vi "pp2_logLoad_trialStringArray.vi"(9 "Input string array":string[](array[string])) -> (2 "Was TRIAL?":bool, 3 "Trial in":T1={"Trial Type Number"=1, "Trial Type"=enum."GO", "Trial Weight"=100, "Shock (mA)"=0.3, "Duration (ms)"=0.25, "Sound Type"=enum."04 FM Sweep", "Stim P1"=4000.0, "Stim P2"=0.0, "Stim P3"=0.0, "Stim P4"=2000.0} {"Shock (mA)" min=-1.0 max=5.0; "Trial Weight" step=1; "Duration (ms)" min=0.0 max=1.0; "Trial Type Number" min=1 max=256 step=1})   [LabVIEW 2013]
uses:
  pp2_CTL_Trial.ctl
  pp2_CTL_TrialType.ctl
  labolabo2/waveforms/WFTypes.ctl
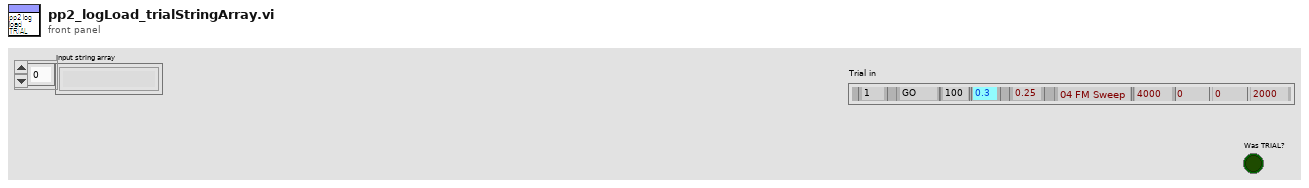
[diagram p1: front panel]
types:
  T1 = typedef "pp2_CTL_Trial.ctl" = cluster{"Trial Type Number":i16, "Trial Type":T2, "Trial Weight":u32, "Shock (mA)":dbl, "Duration (ms)":dbl, "Sound Type":T3, "Stim P1":dbl, "Stim P2":dbl, "Stim P3":dbl, "Stim P4":dbl}
  T2 = typedef "pp2_CTL_TrialType.ctl" = enum16{"OFF", "GO", "NOGO", "TEST"}
  T3 = typedef "WFTypes.ctl" = enum16{"00 NULL", "01 DC", "02 Noise", "03 Pure Tone", "04 FM Sweep"}
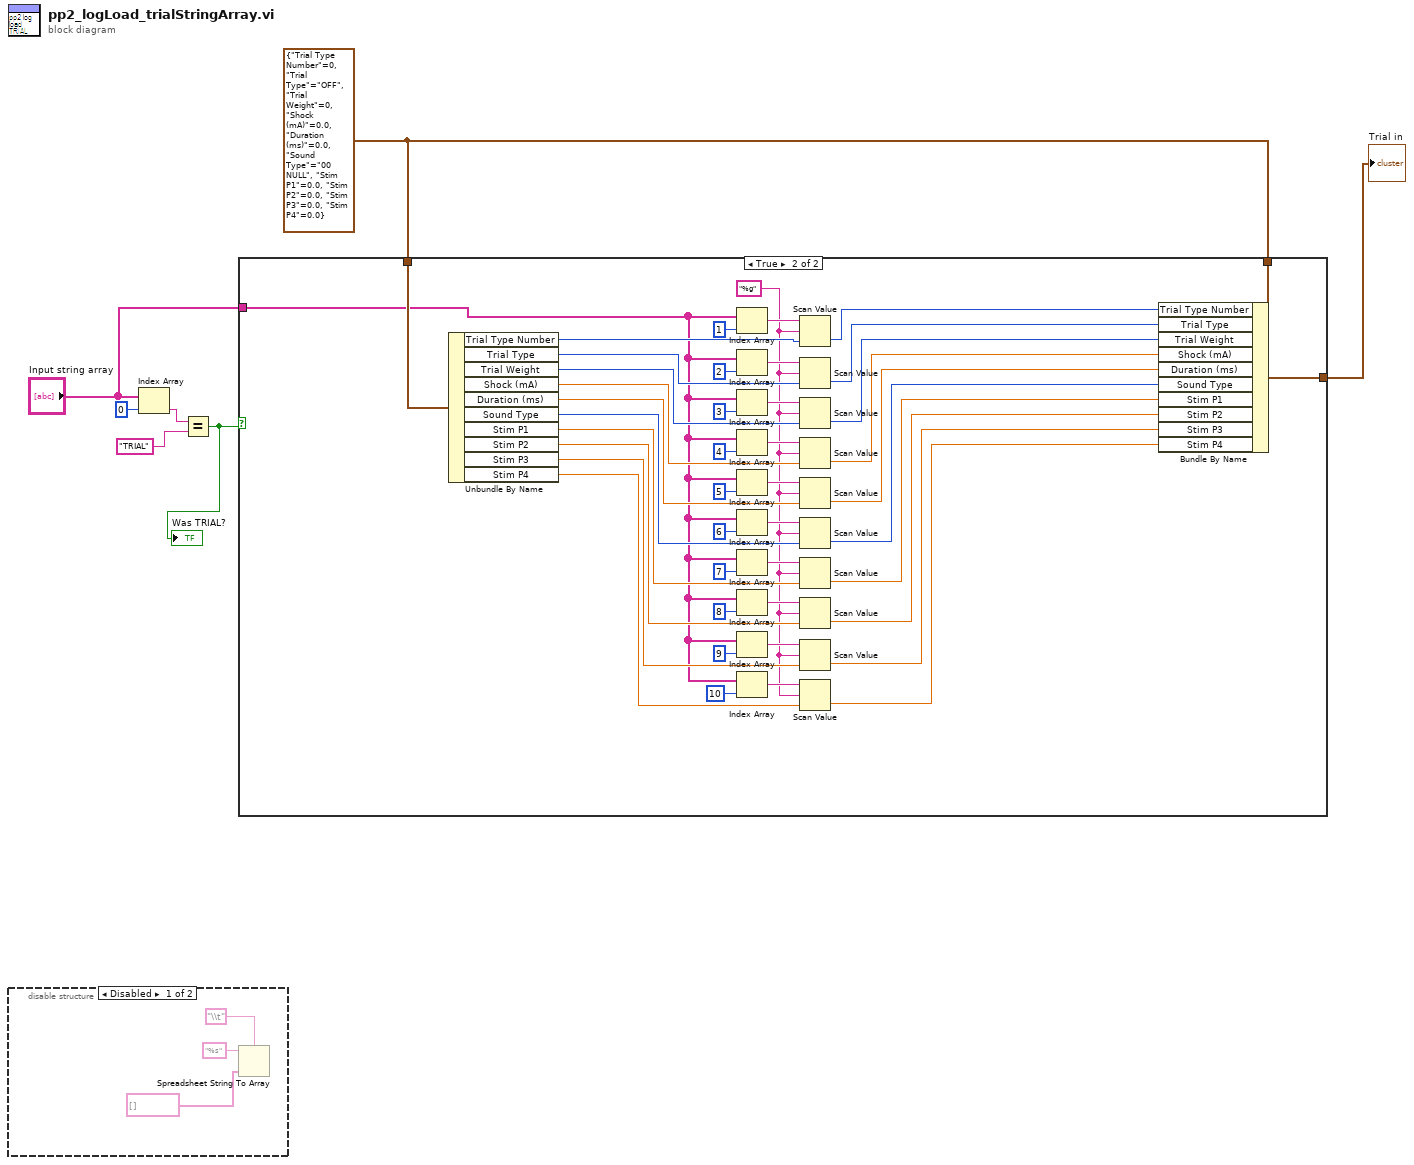
[diagram p0: block diagram]
diagram:
  w2 = T1 {"Trial Type Number"=0, "Trial Type"=enum."OFF", "Trial Weight"=0, "Shock (mA)"=0.0, "Duration (ms)"=0.0, "Sound Type"=enum."00 NULL", "Stim P1"=0.0, "Stim P2"=0.0, "Stim P3"=0.0, "Stim P4"=0.0} ("Trial in")
  n1 = disable-structure shown="Disabled" {
    frame Disabled {
      n2 = Spreadsheet String To Array(delimiter (Tab)="\\t", format string="%s", array type (2D Dbl)=string[] [] ("appended array")) -> (spreadsheet string=w11:string)  [unwired: 1 out]
    }
    frame Enabled {
    }
  }
  n3 = Index Array(array="Input string array", index=0) -> (element=w5:string)
  n4 = Equal?(x=w5, y="TRIAL" ("element")) -> (x = y?=w1:bool)
  "Was TRIAL?" <- w1
  n5 = case shown="True" w1 {
    tunnel: w2 -> [w12 w57]
    tunnel: [w12 w56] -> w7
    tunnel: "Input string array" -> [_ w22]
    tunnel: w2 -> [_ w53]
    frame False {
    }
    frame True {
      w13 = "%g" ("format string")
      n6 = Unbundle By Name(w53) -> ("Trial Type Number"=w51:i16, "Trial Type"=w46:T2, "Trial Weight"=w45:u32, "Shock (mA)"=w36:dbl, "Duration (ms)"=w35:dbl, "Sound Type"=w34:T3, "Stim P1"=w26:dbl, "Stim P2"=w25:dbl, "Stim P3"=w24:dbl, "Stim P4"=w23:dbl)
      n7 = Index Array(array=w22, index=1) -> (element=w54:string)
      n8 = Index Array(array=w22, index=2) -> (element=w49:string)
      n9 = Index Array(array=w22, index=3) -> (element=w47:string)
      n10 = Index Array(array=w22, index=4) -> (element=w41:string)
      n11 = Index Array(array=w22, index=5) -> (element=w39:string)
      n12 = Index Array(array=w22, index=6) -> (element=w37:string)
      n13 = Index Array(array=w22, index=7) -> (element=w14:string)
      n14 = Index Array(array=w22, index=8) -> (element=w31:string)
      n15 = Index Array(array=w22, index=9) -> (element=w29:string)
      n16 = Index Array(array=w22, index=10) -> (element=w27:string)
      n17 = Scan Value(string=w54, format string=w13, default (0 dbl)=w51) -> (value=w52:i16)  [unwired: 1 out]
      n18 = Scan Value(string=w49, format string=w13, default (0 dbl)=w46) -> (value=w44:T2)  [unwired: 1 out]
      n19 = Scan Value(string=w47, format string=w13, default (0 dbl)=w45) -> (value=w43:u32)  [unwired: 1 out]
      n20 = Scan Value(string=w41, format string=w13, default (0 dbl)=w36) -> (value=w21:dbl)  [unwired: 1 out]
      n21 = Scan Value(string=w39, format string=w13, default (0 dbl)=w35) -> (value=w20:dbl)  [unwired: 1 out]
      n22 = Scan Value(string=w37, format string=w13, default (0 dbl)=w34) -> (value=w19:T3)  [unwired: 1 out]
      n23 = Scan Value(string=w14, format string=w13, default (0 dbl)=w26) -> (value=w18:dbl)  [unwired: 1 out]
      n24 = Scan Value(string=w31, format string=w13, default (0 dbl)=w25) -> (value=w17:dbl)  [unwired: 1 out]
      n25 = Scan Value(string=w29, format string=w13, default (0 dbl)=w24) -> (value=w16:dbl)  [unwired: 1 out]
      n26 = Scan Value(string=w27, format string=w13, default (0 dbl)=w23) -> (value=w15:dbl)  [unwired: 1 out]
      n27 = Bundle By Name(cluster=w57, "Trial Type Number"=w52, "Trial Type"=w44, "Trial Weight"=w43, "Shock (mA)"=w21, "Duration (ms)"=w20, "Sound Type"=w19, "Stim P1"=w18, "Stim P2"=w17, "Stim P3"=w16, "Stim P4"=w15) -> (w56:T1)
    }
  }
  "Trial in" <- w7
